vi "Adam_Ch_error_string.vi"(3 "String array":string[](array[string]), 4 "Number of scans":i32) -> (0 "Comment string":string)   [LabVIEW 2010]
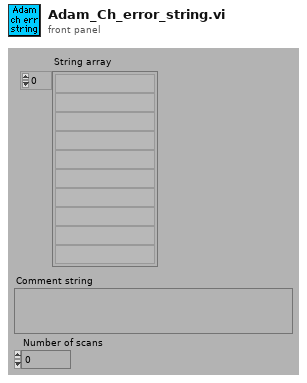
[diagram p1: front panel]
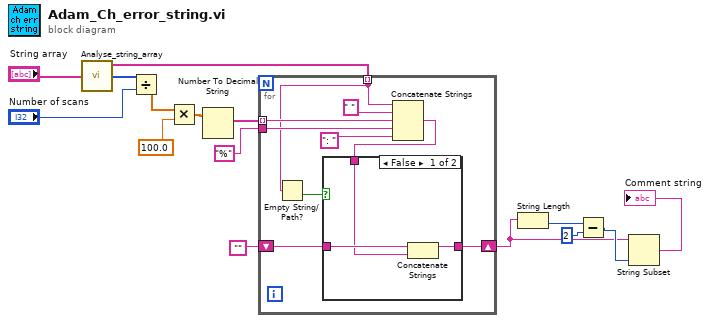
[diagram p0: block diagram]
diagram:
  n1 = call "Analyse_string_array.vi"("String array"="String array") -> ("Unique strings"=w10:string[], "Frequency"=w9:i32[])  [unwired: 1 out]
  n2 = Divide(x=w9, y="Number of scans") -> (x/y=w8:dbl[])
  n3 = Multiply(x=w8, y=100.0) -> (x*y=w13:dbl[])
  n4 = Number To Decimal String(number=w13) -> (decimal integer string=w14:string[])  [unwired: 1 out]
  n5 = for {
    tunnel: w14 -> [w24] mode=indexing
    tunnel: "%" -> [w23]
    tunnel: w10 -> [w21] mode=indexing
    shift-right: [w19] -> w4
    shift-left: "" -> [w18]
    n6 = Empty String/Path?(string/path=w21) -> (empty?=w20:bool)
    n7 = Concatenate Strings(w21, " ", w24, w23, ": ") -> (w17:string)
    n8 = case shown="False" w20 {
      tunnel: [w26 w28] -> w19
      tunnel: w18 -> [w27 w28]
      tunnel: w17 -> [w25 _]
      frame False {
        n9 = Concatenate Strings(w27, w25) -> (w26:string)
      }
      frame True {
      }
    }
  }
  n10 = String Length(string=w4) -> (length=w7:i32)
  n11 = Subtract(x=w7, y=2) -> (x-y=w5:i32)
  n12 = String Subset(string=w4, length (rest)=w5) -> (substring=→"Comment string":string)  [unwired: 1 out]
